vi "Writing-Reading Spreadsheet File.vi"() -> ()   [LabVIEW 2016]
uses:
  <vilib>/Utility/file.llb/Write Delimited Spreadsheet (DBL).vi
  <vilib>/Utility/file.llb/Read Delimited Spreadsheet (DBL).vi
  <vilib>/Waveform/WDTFileIO.llb/ Write Waveform to File.vi
  <vilib>/Waveform/WDTFileIO.llb/Export Waveform To Spreadsheet File.vi
  <vilib>/measure/NI_MABase.lvlib
  <vilib>/measure/NI_MAPro.lvlib
panel:
  in  "Choose the VI pairs to use":T1(ring)
  out "WRITE dt":dbl format="%.2p"
  out "WRITE t0":dbl format="%.3p"
  out "WRITE XY output array":dbl[][](array[numeric]) format="%.3f"
  out "READ dt":sgl format="%.2p"
  out "READ t1":sgl format="%.2p"
  out "READ t0":sgl format="%.3p"
  out "READ Waveform Graph":waveform(dbl)(graph)
  out "WRITE Waveform Graph":waveform(dbl)(graph)
  out "READ Row 1":sgl[](array[numeric]) format="%.3f"
  out "READ Row 0":sgl[](array[numeric]) format="%.3f"
  # "Steps to run:\n1. Select the method of exporting data from LabVIEW to Excel\n2. Run the VI"
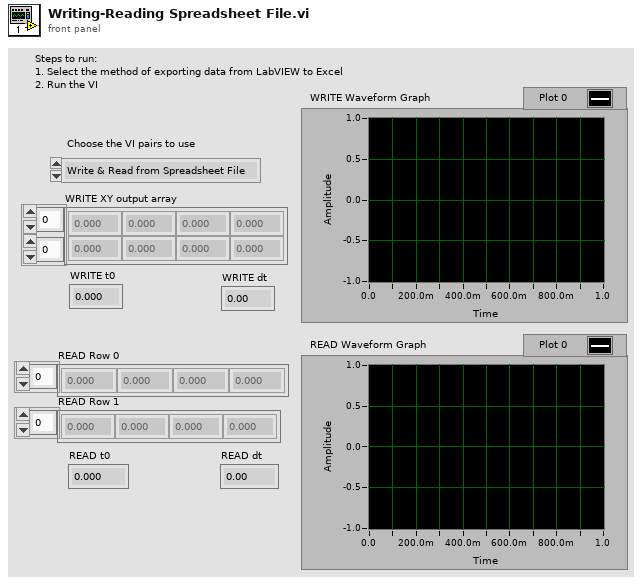
[diagram p1: front panel]
types:
  T1 = enum16{"Write & Read from Spreadsheet File", "Write & Read Waveform from File", "Export & Read Wavefrom from File"}
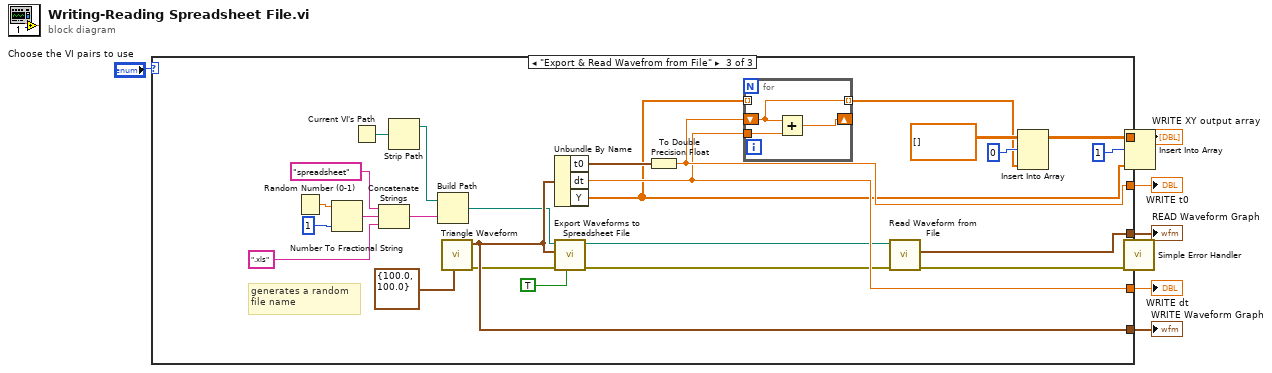
[diagram p0: block diagram]
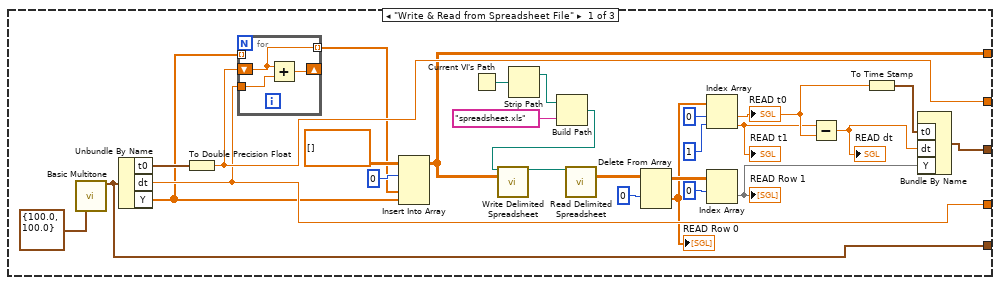
[diagram p2: hidden frame]
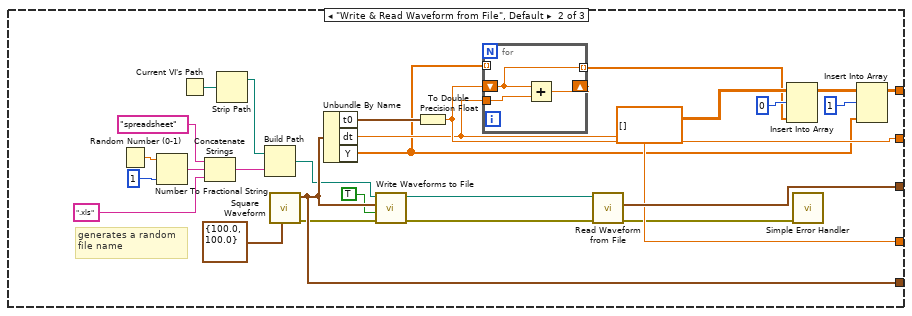
[diagram p3: hidden frame]
diagram:
  n1 = case shown="\"Export & Read Wavefrom from File\"" "Choose the VI pairs to use" {
    tunnel: [w33 w63 w93] -> w5
    tunnel: [w10 w62 w92] -> w4
    tunnel: [w34 w64 w94] -> w3
    tunnel: [w32 w61 w91] -> w2
    tunnel: [w31 w60 w90] -> w1
    frame "Write & Read from Spreadsheet File" {
      n2 = call <vilib>:"Basic Multitone.vi"("sampling info"=cluster{"Fs":dbl, "#s":dbl} {"Fs"=100.0, "#s"=100.0}) -> ("signal out"=w33:waveform(dbl))  [unwired: 11 in, 3 out]
      n3 = Unbundle By Name(w33) -> ("t0"=w21:timestamp, "dt"=w31:dbl, "Y"=w7:dbl[])
      n4 = To Double Precision Float(number=w21) -> (double precision float=w32:dbl)
      n5 = for {
        shift-right: [w36] -> _
        shift-left: w32 -> [w35]
        tunnel: w31 -> [w37]
        tunnel: [w35] -> w26 mode=indexing
        tunnel: w7 -> [_] mode=indexing
        n6 = Add(x=w35, y=w37) -> (x+y=w36:dbl)
      }
      n7 = Insert Into Array "Insert Into Array"(array=dbl[][] [] ("X 2"), index (row)=0, new element #1=w26, new element #2=w7) -> (w10:dbl[][])  [unwired: 1 in]
      n8 = Current VI's Path() -> (path=w23:path)
      n9 = Strip Path(path=w23) -> (stripped path=w22:path)  [unwired: 1 out]
      n10 = Build Path(base path=w22, name or relative path="spreadsheet.xls") -> (appended path=w24:path)
      n11 = call-poly <vilib>:"Write Delimited Spreadsheet.vi"("file path (dialog if empty)"=w24, "2D data"=w10) -> ("new file path (Not A Path if cancelled)"=w30:path)  [unwired: 12 in, 1 out]
      n12 = call-poly <vilib>:"Read Delimited Spreadsheet.vi"("file path (dialog if empty)"=w30) -> ("all rows"=w20:dbl[][])  [unwired: 9 in, 5 out]
      n13 = Delete From Array(array=w20, index (row)=0) -> (deleted portion=w14:dbl[], array with subset deleted=w18:dbl[][])  [unwired: 2 in]
      "READ Row 0" <- w14
      n14 = Index Array(array=w14, index #1=0 ("length"), index #2=1 ("index")) -> (element #1=w16:dbl, element #2=w8:dbl)
      "READ t0" <- w16
      "READ t1" <- w8
      n15 = Index Array(array=w18, index (row)=0) -> (element=w13:dbl[])  [unwired: 1 in]
      "READ Row 1" <- w13
      n16 = Subtract(x=w8, y=w16) -> (x-y=w12:dbl)
      "READ dt" <- w12
      n17 = To Time Stamp(1:w16) -> (0:w11:timestamp)
      n18 = Bundle By Name("t0"=w11, "dt"=w12, "Y"=w13) -> (w34:waveform(dbl))  [unwired: 1 in]
    }
    frame "Write & Read Waveform from File", Default {
      # "generates a random \nfile name"
      n19 = Random Number (0-1)() -> (number: 0 to 1=w46:dbl)
      n20 = Number To Fractional String(number=w46, precision (6)=i16 1) -> (F-format string=w44:string)  [unwired: 2 in]
      n21 = Current VI's Path() -> (path=w49:path)
      n22 = Concatenate Strings("spreadsheet" ("name or relative path"), w44, ".xls" ("string")) -> (w41:string)
      n23 = Strip Path(path=w49) -> (stripped path=w48:path)  [unwired: 1 out]
      n24 = Build Path(base path=w48, name or relative path=w41) -> (appended path=w47:path)
      n25 = call <vilib>:"Square Waveform.vi"("sampling info"=cluster{"Fs":dbl, "#s":dbl} {"Fs"=100.0, "#s"=100.0}) -> ("error out"=w50:errorcluster, "signal out"=w63:waveform(dbl))  [unwired: 9 in]
      n26 = Unbundle By Name(w63) -> ("t0"=w40:timestamp, "dt"=w60:dbl, "Y"=w38:dbl[])
      n27 = call-poly <vilib>:"Write Waveforms to File.vi"("error in (no error)"=w50, "append to file? (new file:F)"=TRUE, "waveform"=w63, "file path (dialog if empty)"=w47) -> ("error out"=w58:errorcluster, "new file path (Not A Path if cancelled)"=w59:path)  [unwired: 6 in]
      n28 = To Double Precision Float(number=w40) -> (double precision float=w61:dbl)
      n29 = for {
        shift-right: [w66] -> _
        shift-left: w61 -> [w65]
        tunnel: w60 -> [w67]
        tunnel: [w65] -> w52 mode=indexing
        tunnel: w38 -> [_] mode=indexing
        n30 = Add(x=w65, y=w67) -> (x+y=w66:dbl)
      }
      n31 = call <vilib>:"Read Waveform from File.vi"("error in (no error)"=w58, "file path (dialog if empty)"=w59) -> ("error out"=w39:errorcluster, "first waveform in record"=w64:waveform(dbl))  [unwired: 4 in, 2 out]
      n32 = Insert Into Array(array=dbl[][] [] ("X 2"), index (row)=0, new element=w52) -> (w54:dbl[][])  [unwired: 1 in]
      n33 = call <vilib>:"Simple Error Handler.vi"("error in (no error)"=w39) -> ()  [unwired: 4 in, 5 out]
      n34 = Insert Into Array(array=w54, index (row)=1, new element=w38) -> (w62:dbl[][])  [unwired: 1 in]
    }
    frame "Export & Read Wavefrom from File" {
      # "generates a random \nfile name"
      n35 = Random Number (0-1)() -> (number: 0 to 1=w76:dbl)
      n36 = Number To Fractional String(number=w76, precision (6)=i16 1) -> (F-format string=w74:string)  [unwired: 2 in]
      n37 = Current VI's Path() -> (path=w79:path)
      n38 = Concatenate Strings("spreadsheet" ("name or relative path"), w74, ".xls" ("string")) -> (w72:string)
      n39 = Strip Path(path=w79) -> (stripped path=w78:path)  [unwired: 1 out]
      n40 = Build Path(base path=w78, name or relative path=w72) -> (appended path=w77:path)
      n41 = call <vilib>:"Triangle Waveform.vi"("sampling info"=cluster{"Fs":dbl, "#s":dbl} {"Fs"=100.0, "#s"=100.0}) -> ("error out"=w80:errorcluster, "signal out"=w93:waveform(dbl))  [unwired: 9 in]
      n42 = Unbundle By Name(w93) -> ("t0"=w70:timestamp, "dt"=w90:dbl, "Y"=w68:dbl[])
      n43 = call-poly <vilib>:"Export Waveforms to Spreadsheet File.vi"("append to file? (new file:F)"=TRUE, "error in (no error)"=w80, "waveform"=w93, "file path (dialog if empty)"=w77) -> ("error out"=w88:errorcluster, "new file path (Not A Path if cancelled)"=w89:path)  [unwired: 6 in]
      n44 = To Double Precision Float(number=w70) -> (double precision float=w91:dbl)
      n45 = for {
        shift-right: [w96] -> _
        shift-left: w91 -> [w95]
        tunnel: w90 -> [w97]
        tunnel: [w95] -> w82 mode=indexing
        tunnel: w68 -> [_] mode=indexing
        n46 = Add(x=w95, y=w97) -> (x+y=w96:dbl)
      }
      n47 = call <vilib>:"Read Waveform from File.vi"("error in (no error)"=w88, "file path (dialog if empty)"=w89) -> ("error out"=w69:errorcluster, "first waveform in record"=w94:waveform(dbl))  [unwired: 4 in, 2 out]
      n48 = Insert Into Array(array=dbl[][] [] ("X 2"), index (row)=0, new element=w82) -> (w84:dbl[][])  [unwired: 1 in]
      n49 = call <vilib>:"Simple Error Handler.vi"("error in (no error)"=w69) -> ()  [unwired: 4 in, 5 out]
      n50 = Insert Into Array(array=w84, index (row)=1, new element=w68) -> (w92:dbl[][])  [unwired: 1 in]
    }
  }
  "WRITE Waveform Graph" <- w5
  "WRITE XY output array" <- w4
  "READ Waveform Graph" <- w3
  "WRITE t0" <- w2
  "WRITE dt" <- w1
